vi "Global_Initialized.vi"() -> ()   [LabVIEW 2019]
panel:
  out "Initialized_Step2?":bool
  out "Initialized_Step1?":bool
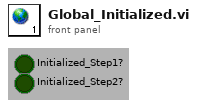
[diagram p1: front panel]
diagram:
